vi "Agilent VNA Read Format.vi"(6 "Channel":i8=1 min=1 max=99 step=1, 7 "Agilent VNA":T1, 8 "error in (no error)":errorcluster, 11 "VISA Resource Name":refnum<visa-resource-name>) -> (0 "error out":errorcluster, 2 "Display Format":T2, 3 "dup VISA Resource Name":refnum<visa-resource-name>)   [LabVIEW 2011]
doc: "This VI for the HP 8753B is used to read the meausurement format.\n\n0 log magnitude\n1 phase\n2 delay\n3 Smith chart\n4 polar\n5 linear magnitude\n6 standing wave ratio\n7 real\n8 imaginary"
uses:
  tests/S Parameter/TypeDefs/SP Measurement Format.ctl
  TypeDefs/Agilent VNA Instrument Info.ctl
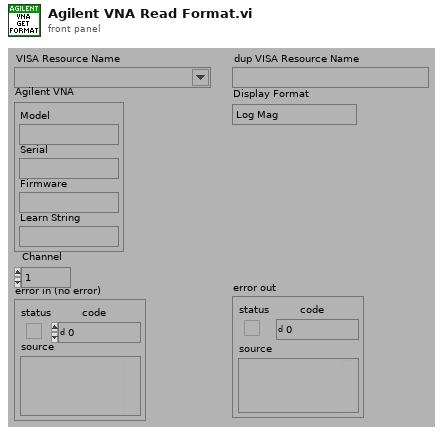
[diagram p1: front panel]
types:
  T1 = typedef "Agilent VNA Instrument Info.ctl" = cluster{"Model":string, "Serial":string, "Firmware":string, "Learn String":string}
  T2 = typedef "SP Measurement Format.ctl" = enum32{"Log Mag", "Phase", "Delay", "Smith (R+jX)", "Polar (Re/Im)", "Linear Mag", "SWR", "Real", "Imaginary", "Smith (Lin/Phase)", "Smith (Log/Phase)", "Smith (Real/Imag)", "Smith (G+jB)", "Polar (Lin/Phase)", "Polar (Log/Phase)", "Expanded Phase", "Positive Phase", "Inverted Smith", "Unwrapped Phase", "Power Out", "Power In", "Linear Mag/Phase", "Log Mag/Phase", "Real/Imaginary"}
  T3 = typedef "Agilent VNA Model.ctl" = enum16{"Not Supported", "8510X", "8719X", "8720X", "8722X", "8753X", "ENA", "PNA", "Field Fox"}
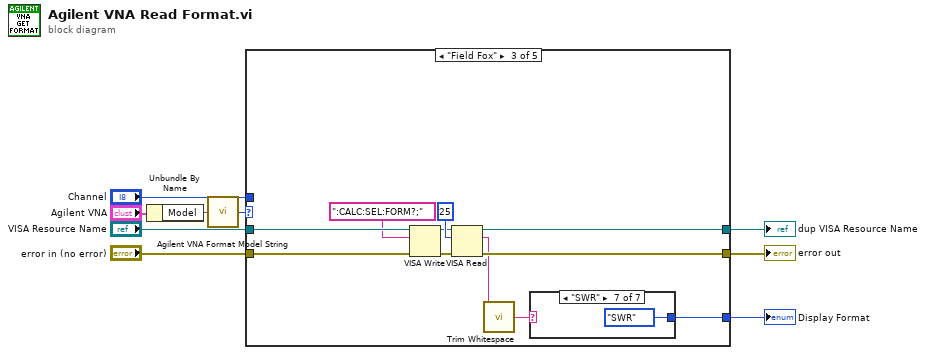
[diagram p0: block diagram]
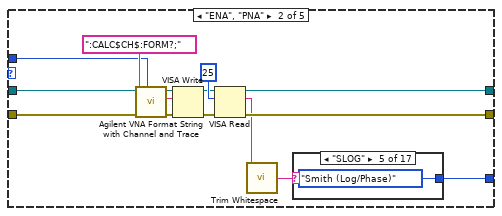
[diagram p3: hidden frame]
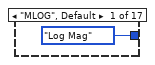
[diagram p4: hidden frame]
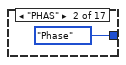
[diagram p5: hidden frame]
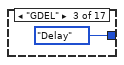
[diagram p6: hidden frame]
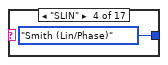
[diagram p7: hidden frame]
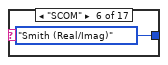
[diagram p8: hidden frame]
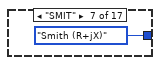
[diagram p9: hidden frame]
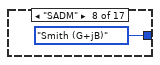
[diagram p10: hidden frame]
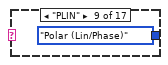
[diagram p11: hidden frame]
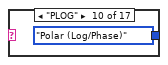
[diagram p12: hidden frame]
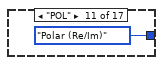
[diagram p13: hidden frame]
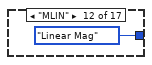
[diagram p14: hidden frame]
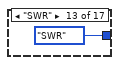
[diagram p15: hidden frame]
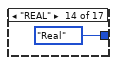
[diagram p16: hidden frame]
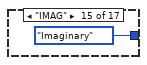
[diagram p17: hidden frame]
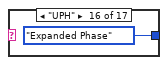
[diagram p18: hidden frame]
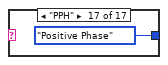
[diagram p19: hidden frame]
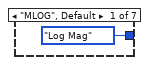
[diagram p20: hidden frame]
diagram:
  n1 = Unbundle By Name("Agilent VNA") -> ("Model"=w1:string)
  n2 = call "Agilent VNA Format Model String.vi"("Model"=w1) -> ("Model"=w4:T3)
  n3 = case shown="\"Field Fox\"" w4 {
    tunnel: "error in (no error)" -> [w10 w18 w46 w70 w102]
    tunnel: [w10 w21 w49 w68 w101] -> w8
    tunnel: [_ w13 w43 w65 w94] -> w7
    tunnel: "VISA Resource Name" -> [w11 w19 w47 w61 w100]
    tunnel: [w11 w20 w48 w60 w99] -> w5
    tunnel: "Channel" -> [_ w12 _ _ _]
    frame "Not Supported" {
    }
    frame "ENA", "PNA" {
      n4 = call "Agilent VNA Format String with Channel and Trace.vi"("Channel"=w12, "String"=":CALC$CH$:FORM?;") -> ("String Out"=w16:string)  [unwired: 1 in, 6 out]
      n5 = VISA Write(VISA resource name=w19, write buffer=w16, error in (no error)=w18) -> (VISA resource name out=w23:refnum<visa-resource-name>, error out=w22:errorcluster)  [unwired: 1 out]
      n6 = VISA Read(VISA resource name=w23, byte count=u32 25, error in (no error)=w22) -> (VISA resource name out=w20:refnum<visa-resource-name>, read buffer=w15:string, error out=w21:errorcluster)  [unwired: 1 out]
      n7 = call <vilib>:"Trim Whitespace.vi"("string"=w15) -> ("trimmed string"=w14:string)  [unwired: 1 in]
      n8 = case shown="\"SLOG\"" w14 {
        tunnel: [SP_Measurement_Format."Log Mag" ("Display Format") SP_Measurement_Format."Phase" ("Display Format") SP_Measurement_Format."Delay" ("Display Format") SP_Measurement_Format."Smith (Lin/Phase)" ("Display Format") SP_Measurement_Format."Smith (Log/Phase)" ("Display Format") SP_Measurement_Format."Smith (Real/Imag)" ("Display Format") SP_Measurement_Format."Smith (R+jX)" ("Display Format") SP_Measurement_Format."Smith (G+jB)" ("Display Format") SP_Measurement_Format."Polar (Lin/Phase)" ("Display Format") SP_Measurement_Format."Polar (Log/Phase)" ("Display Format") SP_Measurement_Format."Polar (Re/Im)" ("Display Format") SP_Measurement_Format."Linear Mag" ("Display Format") SP_Measurement_Format."SWR" ("Display Format") SP_Measurement_Format."Real" ("Display Format") SP_Measurement_Format."Imaginary" ("Display Format") SP_Measurement_Format."Expanded Phase" ("Display Format") SP_Measurement_Format."Positive Phase" ("Display Format")] -> w13
        frame "MLOG", Default {
        }
        frame "PHAS" {
        }
        frame "GDEL" {
        }
        frame "SLIN" {
        }
        frame "SLOG" {
        }
        frame "SCOM" {
        }
        frame "SMIT" {
        }
        frame "SADM" {
        }
        frame "PLIN" {
        }
        frame "PLOG" {
        }
        frame "POL" {
        }
        frame "MLIN" {
        }
        frame "SWR" {
        }
        frame "REAL" {
        }
        frame "IMAG" {
        }
        frame "UPH" {
        }
        frame "PPH" {
        }
      }
    }
    frame "Field Fox" {
      n9 = VISA Write(VISA resource name=w47, write buffer=":CALC:SEL:FORM?;", error in (no error)=w46) -> (VISA resource name out=w51:refnum<visa-resource-name>, error out=w50:errorcluster)  [unwired: 1 out]
      n10 = VISA Read(VISA resource name=w51, byte count=u32 25, error in (no error)=w50) -> (VISA resource name out=w48:refnum<visa-resource-name>, read buffer=w45:string, error out=w49:errorcluster)  [unwired: 1 out]
      n11 = call <vilib>:"Trim Whitespace.vi"("string"=w45) -> ("trimmed string"=w44:string)  [unwired: 1 in]
      n12 = case shown="\"SWR\"" w44 {
        tunnel: [SP_Measurement_Format."Log Mag" ("Display Format") SP_Measurement_Format."Phase" ("Display Format") SP_Measurement_Format."Delay" ("Display Format") SP_Measurement_Format."Smith (R+jX)" ("Display Format") SP_Measurement_Format."Polar (Re/Im)" ("Display Format") SP_Measurement_Format."Linear Mag" ("Display Format") SP_Measurement_Format."SWR" ("Display Format")] -> w43
        frame "MLOG", Default {
        }
        frame "PHAS" {
        }
        frame "GDEL" {
        }
        frame "SMIT" {
        }
        frame "POL" {
        }
        frame "MLIN" {
        }
        frame "SWR" {
        }
      }
    }
    frame "8719X".."8753X" {
      w62 = string[] ["LOGM", "PHAS", "DELA", "SMIC", "POLA", "LINM", "SWR", "REAL", "IMAG"]
      n13 = Array Size(array=w62) -> (size(s)=w69:i32)
      n14 = Decrement(x=w69) -> (x-1=w64:i32)
      n15 = while {
        tunnel: w61 -> [w87]
        shift-right: [w78] -> w68
        shift-left: w70 -> [w79]
        tunnel: w62 -> [w80] mode=indexing
        tunnel: w64 -> [w77]
        tunnel: [w71] -> w63
        tunnel: [w72] -> w60
        i -> [w71]
        stop <- w73 stop-if-true
        n16 = Concatenate Strings(w80, "?;") -> (w81:string)
        n17 = VISA Write(VISA resource name=w87, write buffer=w81, error in (no error)=w79) -> (VISA resource name out=w88:refnum<visa-resource-name>, error out=w90:errorcluster)  [unwired: 1 out]
        n18 = VISA Read(VISA resource name=w88, byte count=u32 25, error in (no error)=w90) -> (VISA resource name out=w72:refnum<visa-resource-name>, read buffer=w85:string, error out=w78:errorcluster)  [unwired: 1 out]
        n19 = Fract/Exp String To Number(use system decimal point (T)=FALSE, string=w85) -> (number=w86:dbl)  [unwired: 3 out]
        n20 = Equal?(x=w77, y=w71) -> (x = y?=w76:bool)
        n21 = To Unsigned Long Integer(number=w86) -> (unsigned 32bit integer=w83:u32)
        n22 = Unbundle(w78) -> ("status"=w75:bool)  [unwired: 2 out]
        n23 = Not Equal To 0?(x=w83) -> (x != 0?=w74:bool)
        n24 = Compound Arithmetic op=OR(w74, w75, w76) -> (w73:bool)
      }
      n25 = To Unsigned Long Integer(number=w63) -> (unsigned 32bit integer=w67:u32)
      n26 = Type Cast(type=SP_Measurement_Format."Log Mag" ("Display Format"), x=w67) -> (*(type *) &x=w65:T2)
    }
    frame "8510X" {
      n27 = VISA Write(VISA resource name=w100, write buffer="FORM?;", error in (no error)=w102) -> (VISA resource name out=w96:refnum<visa-resource-name>, error out=w98:errorcluster)  [unwired: 1 out]
      n28 = VISA Read(VISA resource name=w96, byte count=u32 25, error in (no error)=w98) -> (VISA resource name out=w99:refnum<visa-resource-name>, read buffer=w92:string, error out=w101:errorcluster)  [unwired: 1 out]
      n29 = call <vilib>:"Trim Whitespace.vi"("string"=w92) -> ("trimmed string"=w93:string)  [unwired: 1 in]
      n30 = call "Strip Quotes From String.vi"("String In"=w93) -> ("Trimmed String"=w91:string)
      n31 = case shown="\"LOG MAG\", Default" w91 {
        tunnel: [SP_Measurement_Format."Log Mag" ("Display Format") SP_Measurement_Format."Phase" ("Display Format") SP_Measurement_Format."Delay" ("Display Format") SP_Measurement_Format."Smith (R+jX)" ("Display Format") SP_Measurement_Format."SWR" ("Display Format") SP_Measurement_Format."Linear Mag" ("Display Format") SP_Measurement_Format."Polar (Lin/Phase)" ("Display Format") SP_Measurement_Format."Polar (Log/Phase)" ("Display Format") SP_Measurement_Format."Polar (Re/Im)" ("Display Format") SP_Measurement_Format."Inverted Smith" ("Display Format") SP_Measurement_Format."Imaginary" ("Display Format") SP_Measurement_Format."Real" ("Display Format")] -> w94
        frame "LOG MAG", Default {
        }
        frame "PHASE" {
        }
        frame "DELAY" {
        }
        frame "SMITH CHART" {
        }
        frame "SWR" {
        }
        frame "LINEAR MAGNITUDE" {
        }
        frame "LIN mkr on POLAR" {
        }
        frame "LOG mkr on POLAR" {
        }
        frame "Re/Im mkr on POLAR" {
        }
        frame "INVERTED SMITH" {
        }
        frame "IMAGINARY" {
        }
        frame "REAL" {
        }
      }
    }
  }
  "Display Format" <- w7
  "dup VISA Resource Name" <- w5
  "error out" <- w8
